vi "ArmGetXYZ.vi"() -> (1 "GetZ":dbl, 2 "GetY":dbl, 3 "GetX":dbl)   [LabVIEW 2020]
doc: "Get XYZ from arm globals\n\nOutputs:\n--X--Double\n--Y--Double\n--Z--Double"
uses:
  ArmGlobal.vi
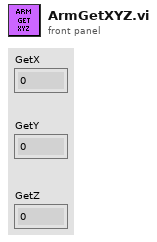
[diagram p1: front panel]
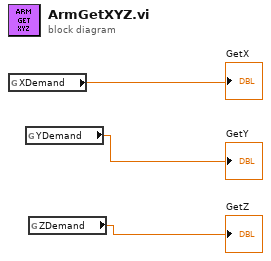
[diagram p0: block diagram]
diagram:
  n1 = global read "ArmGlobal.vi" "XDemand"() -> (→"GetX":dbl)
  n2 = global read "ArmGlobal.vi" "YDemand"() -> (→"GetY":dbl)
  n3 = global read "ArmGlobal.vi" "ZDemand"() -> (→"GetZ":dbl)
